vi "Joystick Toggle.vi"(4 "Max":dbl, 6 "Min":dbl, 9 "Value":dbl, 11 "Range":dbl) -> (1 "Output":dbl)   [LabVIEW 2018]
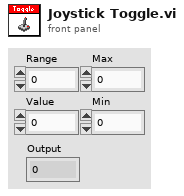
[diagram p1: front panel]
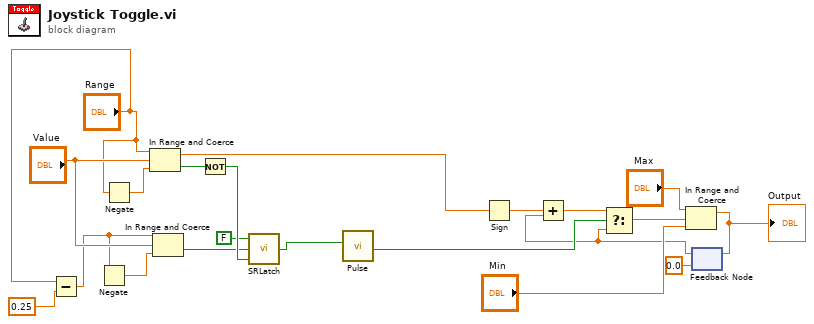
[diagram p0: block diagram]
diagram:
  n1 = Subtract(x="Range", y=0.25) -> (x-y=w1:dbl)
  n2 = Negate(x=w1) -> (-x=w9:dbl)
  n3 = Negate(x="Range") -> (-x=w20:dbl)
  n4 = In Range and Coerce(upper limit="Range", x="Value", lower limit=w20) -> (coerced(x)=w16:dbl, In Range?=w21:bool)
  n5 = In Range and Coerce(upper limit=w1, x="Value", lower limit=w9) -> (In Range?=w6:bool)  [unwired: 1 out]
  n6 = Not(x=w21) -> (.not. x?=w8:bool)
  n7 = call "SRLatch.vi"("On"=w8, "Off"=w6, "Initial"=FALSE) -> ("Output"=w7:bool)
  n8 = call "Pulse.vi"("Input"=w7) -> ("Output"=w18:bool)  [unwired: 10 in]
  n9 = Sign(1:w16) -> (0:w19:dbl)
  n10 = feedback #1(0.0 ("Max")) -> (w11:dbl)
  n11 = Add(x=w19, y=w11) -> (x+y=w17:dbl)
  n12 = Select(t=w17, s=w18, f=w11) -> (s? t:f=w15:dbl)
  n13 = In Range and Coerce(upper limit="Max", x=w15, lower limit="Min") -> (coerced(x)=w12:dbl)  [unwired: 1 out]
  "Output" <- w12
  n14 = feedback-in #1(w12) -> ()
